vi "Event Handler.vi"(8 "error in (no error)":errorcluster, 10 "Stop Event Handler":refnum<user-event>, 11 "PhoneFromField in":refnum<class "PhoneFromField.lvclass">) -> (0 "error out":errorcluster)   [LabVIEW 2019, in "PhoneFromField.lvclass"]
doc: "The <b>Event Handler VI</b> is a dynamic dispatch VI that should be overwritten if events are needed to create the enhanced QControl. \n\nBy inheriting from the main Control.lvclass the overwritten <b>Event Handler VI</b> will be launched asynchronously in the initialization of the QControl.\n<b> </b> <b> </b>\n©2016 Q Software Innovations, LLC (QSI)\nwritten by Quentin Alldredge\nproduced in LabVIEW 2015\n\nsupport@qsoftwareinnovations.com\nwww.qsoftwareinnovations.com\n\nAll rights reserved.\n\nRedistribution and use in source and binary forms, with or without modification, are permitted provided that the following conditions are met:\n\n * Redistributions of source code must retain the above copyright notice, this list of conditions and the following disclaimer.\n * Redistributions in binary form must reproduce the above copyright notice, this list of conditions and the following disclaimer in the documentation and/or other materials provided with the distribution.\n * Neither the name of Q Software Innovations, LLC. nor the names of its contributors may be used to endorse or promote products derived from this software without specific prior written permission.\n\nTHIS SOFTWARE IS PROVIDED BY THE COPYRIGHT HOLDERS AND CONTRIBUTORS \"AS IS\" AND ANY EXPRESS OR IMPLIED WARRANTIES, INCLUDING, BUT NOT LIMITED TO, THE IMPLIED WARRANTIES OF MERCHANTABILITY AND FITNESS FOR A PARTICULAR PURPOSE ARE DISCLAIMED. IN NO EVENT SHALL THE COPYRIGHT OWNER OR CONTRIBUTORS BE LIABLE FOR ANY DIRECT, INDIRECT, INCIDENTAL, SPECIAL, EXEMPLARY, OR CONSEQUENTIAL DAMAGES (INCLUDING, BUT NOT LIMITED TO, PROCUREMENT OF SUBSTITUTE GOODS OR SERVICES; LOSS OF USE, DATA, OR PROFITS; OR BUSINESS INTERRUPTION) HOWEVER CAUSED AND ON ANY THEORY OF LIABILITY, WHETHER IN CONTRACT, STRICT LIABILITY, OR TORT (INCLUDING NEGLIGENCE OR OTHERWISE) ARISING IN ANY WAY OUT OF THE USE OF THIS SOFTWARE, EVEN IF ADVISED OF THE POSSIBILITY OF SUCH DAMAGE."
uses:
  PhoneFromField.lvclass
  C:/Program Files (x86)/National Instruments/LabVIEW 2019/vi.lib/QSI/QControls/QControl Classes/String/String.lvclass
  PhoneFromField.lvclass/PhoneFromField.ctl
  <vilib>/regexp/Match Regular Expression.xnode
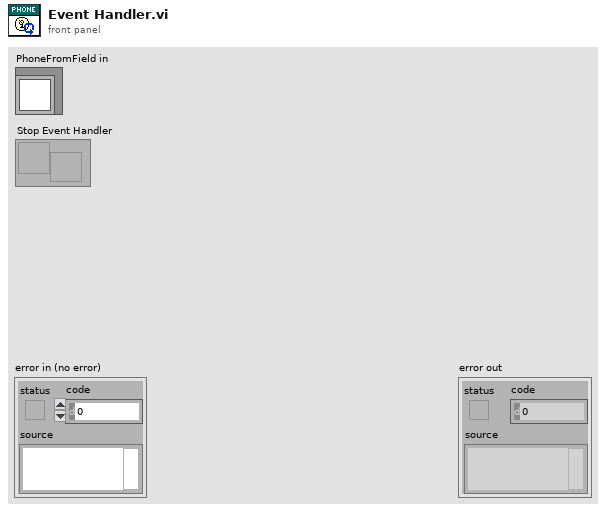
[diagram p1: front panel]
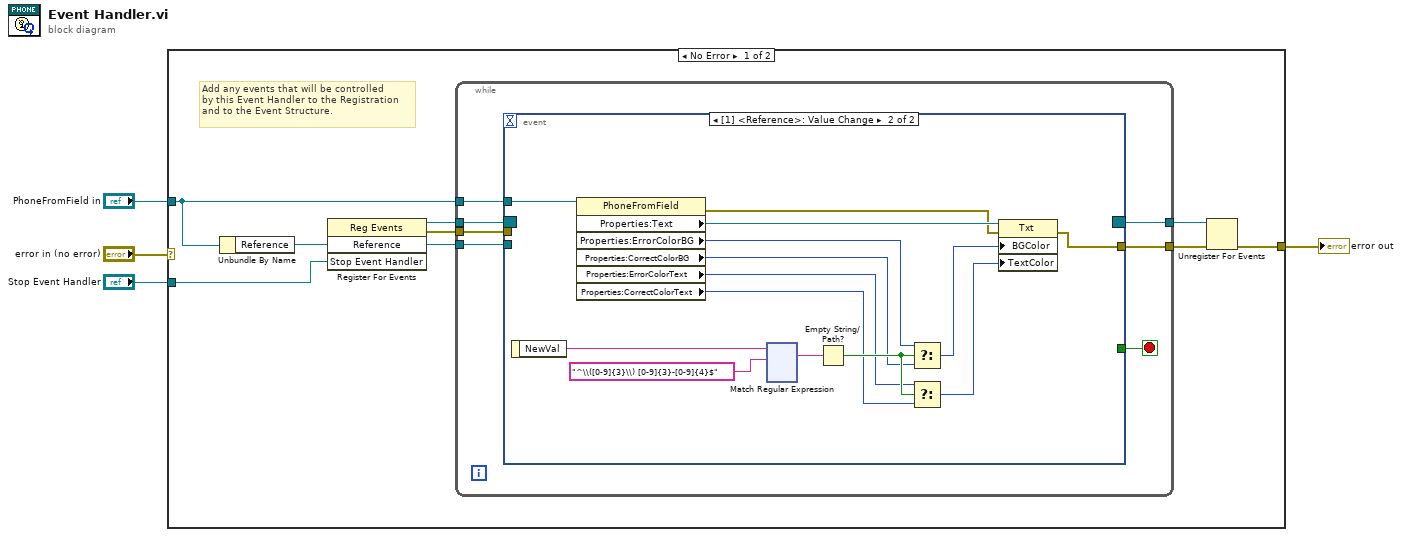
[diagram p0: block diagram]
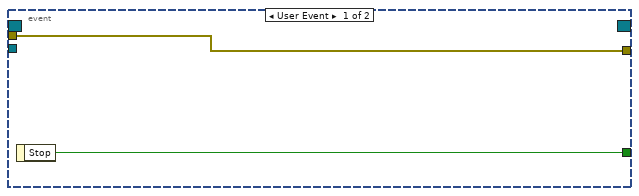
[diagram p2: hidden frame]
diagram:
  n1 = case shown="No Error" "error in (no error)" {
    selector: "error in (no error)" -> [_ w150]
    tunnel: [w9 w150] -> w3
    tunnel: "PhoneFromField in" -> [w7 _]
    tunnel: "Stop Event Handler" -> [w5 _]
    frame No Error {
      # "Add any events that will be controlled\nby this Event Handler to the Registration\nand to the Event Structure."
      n2 = Unbundle By Name(w7) -> ("Reference"=w6:refnum<vi>)
      n3 = register-events(w6, w5) -> (reference out=w12:refnum<event-registration>, error out=w11:errorcluster)  [unwired: 2 in]
      n4 = while {
        tunnel: w12 -> [w19]
        tunnel: w11 -> [w17]
        tunnel: [w16] -> w10
        tunnel: [w14] -> w8
        tunnel: w6 -> [w13]
        tunnel: w7 -> [w18]
        stop <- w15 stop-if-true
        n5 = event shown="[1] <Reference>: Value Change" {
          selector: w19 -> [_ _]
          dyn-events: [_ _] -> w14
          timeout: _ -> [_ _]
          tunnel: w18 -> [_ w35]
          tunnel: w17 -> [w21 _]
          tunnel: [w21 w27] -> w16
          tunnel: [w20 _] -> w15
          tunnel: w13 -> [_ _]
          event User Event {
            n6 = event-data() -> ("Stop"=w20:bool)  [unwired: 1 in]
          }
          event Value Change {
            n7 = event-data() -> ("NewVal"=w34:string)  [unwired: 1 in]
            n8 = property class="PhoneFromField"(reference=w35) -> (error out=w28:errorcluster, "Properties:Text"=w31:refnum<vi>, "Properties:ErrorColorBG"=w25:u32, "Properties:CorrectColorBG"=w24:u32, "Properties:ErrorColorText"=w23:u32, "Properties:CorrectColorText"=w22:u32)  [unwired: 1 in, 1 out]
            n9 = xnode "Match Regular Expression"("input string"=w34, "regular expression"="^\\([0-9]{3}\\) [0-9]{3}-[0-9]{4}$") -> ("whole match"=w32:string)  [unwired: 4 in, 4 out]
            n10 = Empty String/Path?(string/path=w32) -> (empty?=w29:bool)
            n11 = Select(t=w25, s=w29, f=w24) -> (s? t:f=w30:u32)
            n12 = Select(t=w23, s=w29, f=w22) -> (s? t:f=w26:u32)
            n13 = property class="Txt"(reference=w31, error in=w28, "BGColor"=w30, "TextColor"=w26) -> (error out=w27:errorcluster)  [unwired: 1 out]
          }
        }
      }
      n14 = Unregister For Events(event registration refnum=w8, error in=w10) -> (error out=w9:errorcluster)
    }
    frame Error {
    }
  }
  "error out" <- w3
